vi "New Worker UI.vi"(11 "Starting Name":string) -> (0 "New Project?":bool, 1 "Project":refnum<vi>, 2 "Cancelled?":bool, 3 "New Name":string, 4 "Selected Actions":T1)   [LabVIEW 2022 SP3, in "FlexBlocks Support.lvlib"]
uses:
  FlexBlocks Support.lvlib
  Action Selections.ctl
panel:
  out "Action Diagram":picture
  out "Action Name":string
  out "Info":string
  in  "Actions":T1
  in  "Project Select":string(combo)
  in  "Add To Project":bool
  in  "Cancel":bool
  in  "OK":bool
  # "Enter the name of the new Worker to create:"
  # "Mouseover actions for descriptions."
  # "Unselected actions can later be added to workers by adding the specific case selection back in the Work.vi"
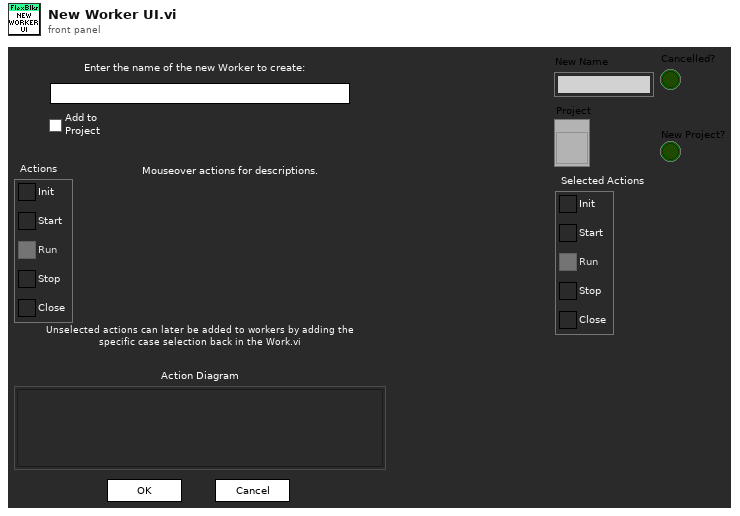
[diagram p1: front panel]
types:
  T1 = typedef "FlexBlocks Support.lvlib/Action Selections.ctl" = cluster{"Init":bool, "Start":bool, "Run":bool, "Stop":bool, "Close":bool}
  T2 = cluster{"Init":bool, "Start":bool, "Run":bool, "Stop":bool, "Close":bool}
  T3 = typedef "FlexBlocks Support.lvlib/Paths.ctl" = cluster{"FlexBlocks":path, "Workers Root":path, "Specialized Editors":path, "Worker Template":path, "SM Template":path, "Read Control Value Vim":path, "Write Indicator Value Vim":path}
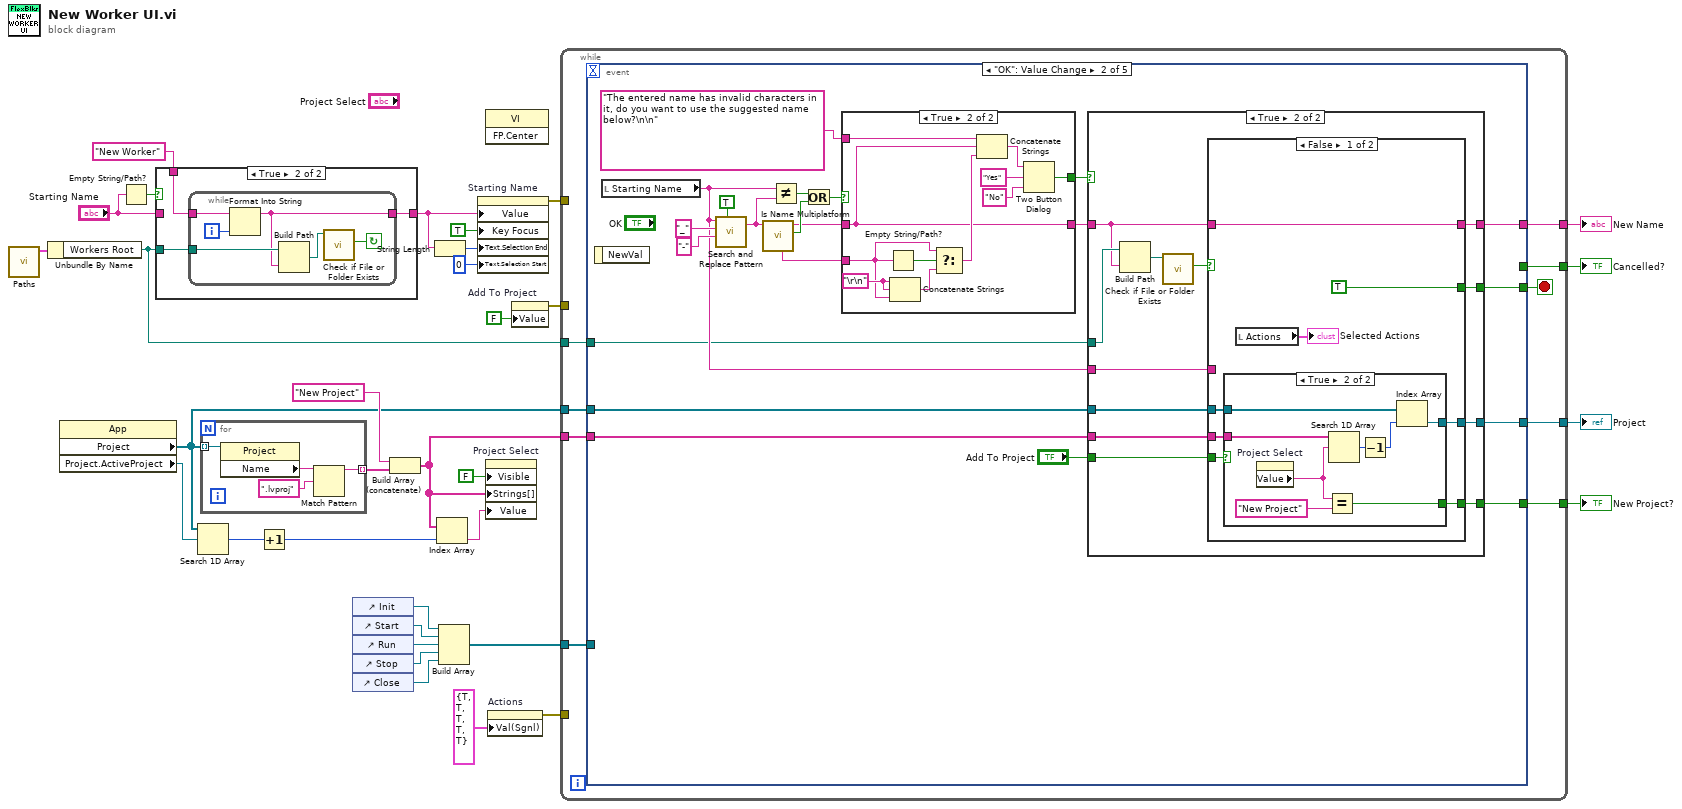
[diagram p0: block diagram]
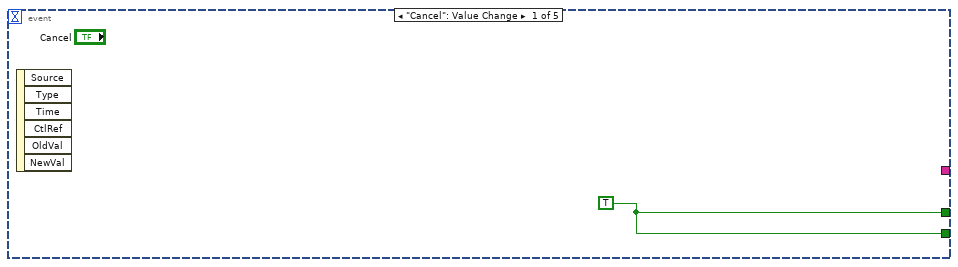
[diagram p2: hidden frame]
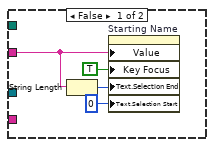
[diagram p3: hidden frame]
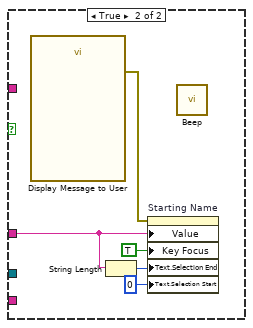
[diagram p5: hidden frame]
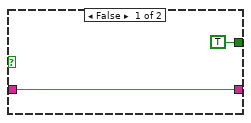
[diagram p6: hidden frame]
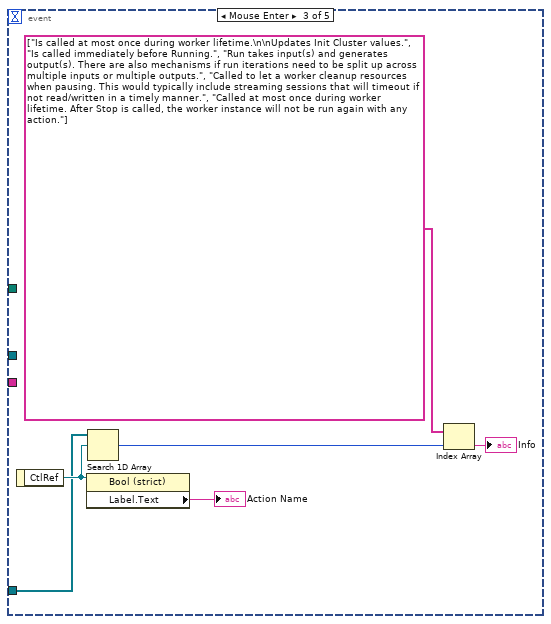
[diagram p7: hidden frame]
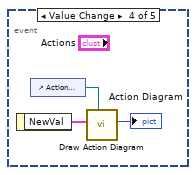
[diagram p8: hidden frame]
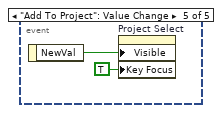
[diagram p9: hidden frame]
diagram:
  n1 = call "Paths.vi"() -> ("Paths"=w18:T3)  [unwired: 11 in]
  n2 = Unbundle By Name(w18) -> ("Workers Root"=w9:path)
  n3 = property class="App"() -> ("Project"=w15:refnum<vi>[], "Project.ActiveProject"=w24:refnum<vi>)  [unwired: 2 in, 2 out]
  n4 = Empty String/Path?(string/path="Starting Name") -> (empty?=w31:bool)
  n5 = case shown="True" w31 {
    tunnel: "Starting Name" -> [w34 _]
    tunnel: w9 -> [_ w37]
    tunnel: [w34 w36] -> w27
    tunnel: "New Worker" -> [_ w35]
    frame False {
    }
    frame True {
      n6 = while {
        tunnel: w37 -> [w42]
        tunnel: [w39] -> w36
        tunnel: w35 -> [w38]
        i -> [w43]
        stop <- w40 continue-if-true
        n7 = Format Into String(initial string=w38, w43) -> (resulting string=w39:string)  [unwired: 2 in, 1 out]
        n8 = Build Path(base path=w42, name or relative path=w39) -> (appended path=w41:path)
        n9 = call <vilib>:"Check if File or Folder Exists.vi"("path"=w41) -> ("file or folder exists?"=w40:bool)  [unwired: 8 in, 2 out]
      }
    }
  }
  n10 = Search 1D Array(1D array=w15, element=w24) -> (index of element=w23:i32)  [unwired: 1 in]
  n11 = for {
    tunnel: w15 -> [w47] mode=indexing
    tunnel: [w44] -> w21 mode=indexing
    n12 = property class="Project"(reference=w47) -> ("Name"=w46:string)  [unwired: 1 in, 2 out]
    n13 = Match Pattern(string=w46, regular expression=".lvproj") -> (before substring=w44:string)  [unwired: 1 in, 3 out]
  }
  n14 = Increment(x=w23) -> (x+1=w19:i32)
  n15 = control-ref of="Init"() -> (w4:refnum<vi>)
  n16 = control-ref of="Start"() -> (w5:refnum<vi>)
  n17 = control-ref of="Run"() -> (w8:refnum<vi>)
  n18 = control-ref of="Stop"() -> (w7:refnum<vi>)
  n19 = control-ref of="Close"() -> (w6:refnum<vi>)
  n20 = Build Array (concatenate)("New Project", w21) -> (w14:string[])
  n21 = String Length(string=w27) -> (length=w29:i32)
  n22 = Index Array(array=w14, index=w19) -> (element=w22:string)
  n23 = Build Array(w4, w5, w8, w7, w6) -> (w3:refnum<vi>[])
  n24 = property on="Starting Name" class="Str"("Value"=w27, "Key Focus"=TRUE, "Text.Selection End"=w29, "Text.Selection Start"=u32 0 ("Text.Selection:Start")) -> (error out=w17:errorcluster)  [unwired: 2 in, 1 out]
  n25 = invoke class="VI" method="FP.Center"() -> ()  [unwired: 3 in, 3 out]
  n26 = property on="Project Select" class="CmbBox"("Visible"=FALSE, "Strings[]"=w14, "Value"=w22) -> ()  [unwired: 2 in, 2 out]
  n27 = property on="Actions" class="Clust (strict)"("Val(Sgnl)"=T2 {"Init"=TRUE, "Start"=TRUE, "Run"=TRUE, "Stop"=TRUE, "Close"=TRUE} ("Value (Signaling)")) -> (error out=w2:errorcluster)  [unwired: 2 in, 1 out]
  n28 = property on="Add To Project" class="Bool (strict)"("Value"=FALSE ("Add To Project")) -> (error out=w16:errorcluster)  [unwired: 2 in, 1 out]
  n29 = while {
    tunnel: w17 -> [_]
    tunnel: w16 -> [_]
    tunnel: w15 -> [w53]
    tunnel: w14 -> [w52]
    tunnel: [w55] -> w13
    tunnel: [w54] -> w12
    tunnel: [w51] -> w11
    tunnel: [w50] -> w10
    tunnel: w9 -> [w49]
    tunnel: w3 -> [w48]
    tunnel: w2 -> [_]
    stop <- w56 stop-if-true
    n30 = event shown="[1] \"OK\": Value Change" {
      selector: _ -> [_ _ _ _ _]
      dyn-events: _ -> [_ _ _ _ _]
      timeout: _ -> [_ _ _ _ _]
      tunnel: [w57 w61 _ _ _] -> w56
      tunnel: [w57 _ _ _ _] -> w55
      tunnel: [_ w65 _ _ _] -> w54
      tunnel: w53 -> [_ w64 _ _ _]
      tunnel: w52 -> [_ w63 _ _ _]
      tunnel: [_ w62 _ _ _] -> w51
      tunnel: [_ w60 _ _ _] -> w50
      tunnel: w49 -> [_ w58 _ _ _]
      tunnel: w48 -> [_ _ w132 _ _]
      event "Cancel": Value Change {
        w57 = TRUE
        n31 = event-data() -> ()  [unwired: 1 in, 6 out]
      }
      event "OK": Value Change {
        n32 = event-data() -> ()  [unwired: 1 in, 1 out]
        n33 = local read "Starting Name"() -> (w59:string)
        n34 = call <vilib>:"Search and Replace Pattern.vi"("string"=w59, "regular expression (\"\")"="_" ("regular expression (\"\")"), "replace string (\"\")"="-" ("replace string (\"\")"), "replace all? (F)"=TRUE) -> ("result string"=w72:string)  [unwired: 1 in, 1 out]
        n35 = call <vilib>:"Is Name Multiplatform.vi"("filename"=w72) -> ("filename had conflict"=w77:bool, "suggested filename"=w76:string, "problem description"=w78:string)  [unwired: 6 in, 2 out]
        n36 = Not Equal?(x=w59, y=w72) -> (x != y?=w70:bool)
        n37 = Or(x=w70, y=w77) -> (x .or. y?=w71:bool)
        n38 = case shown="True" w71 {
          tunnel: w78 -> [_ w122]
          tunnel: w76 -> [w117 w118]
          tunnel: "The entered name has invalid characters in it, do you want to use the suggested name below?\n\n" -> [_ w126]
          tunnel: [TRUE ("T button?") w119] -> w67
          tunnel: [w117 w118] -> w68
          frame False {
          }
          frame True {
            w124 = "\r\n"
            n39 = Empty String/Path?(string/path=w122) -> (empty?=w125:bool)
            n40 = Concatenate Strings(w124, w124, w122) -> (w123:string)
            n41 = Select(t=w122, s=w125, f=w123) -> (s? t:f=w121:string)
            n42 = Concatenate Strings(w126, w118, w121) -> (w120:string)
            n43 = Two Button Dialog(message=w120, 1:"No" ("F button name (\"Cancel\")"), 2:"Yes" ("T button name (\"OK\")")) -> (T button?=w119:bool)
          }
        }
        n44 = case shown="True" w67 {
          tunnel: w68 -> [_ w90]
          tunnel: w58 -> [_ w94]
          tunnel: [_ w91] -> w61
          tunnel: [_ w89] -> w60
          tunnel: w59 -> [w79 w88]
          tunnel: w63 -> [_ w87]
          tunnel: w64 -> [_ w86]
          tunnel: "Add To Project" -> [_ w85]
          tunnel: [_ w84] -> w62
          tunnel: [_ w83] -> w65
          frame False {
            n45 = String Length(string=w79) -> (length=w82:i32)
            n46 = property on="Starting Name" class="Str"("Value"=w79, "Key Focus"=TRUE, "Text.Selection End"=w82, "Text.Selection Start"=u32 0 ("Text.Selection:Start")) -> ()  [unwired: 2 in, 2 out]
          }
          frame True {
            n47 = Build Path(base path=w94, name or relative path=w90) -> (appended path=w93:path)
            n48 = call <vilib>:"Check if File or Folder Exists.vi"("path"=w93) -> ("file or folder exists?"=w92:bool)  [unwired: 8 in, 2 out]
            n49 = case shown="False" w92 {
              tunnel: [TRUE _] -> w91
              tunnel: w90 -> [w101 _]
              tunnel: [w101 _] -> w89
              tunnel: w88 -> [_ w111]
              tunnel: w87 -> [w99 _]
              tunnel: w86 -> [w98 _]
              tunnel: w85 -> [w100 _]
              tunnel: [w97 _] -> w84
              tunnel: [w96 _] -> w83
              frame False {
                n50 = case shown="True" w100 {
                  tunnel: w99 -> [_ w110]
                  tunnel: w98 -> [_ w109]
                  tunnel: [_ w107] -> w97
                  tunnel: [_ w104] -> w96
                  frame False {
                  }
                  frame True {
                    n51 = property on="Project Select" class="CmbBox"() -> ("Value"=w106:string)  [unwired: 2 in, 2 out]
                    n52 = Equal?(x=w106, y="New Project") -> (x = y?=w104:bool)
                    n53 = Search 1D Array(1D array=w110, element=w106) -> (index of element=w108:i32)  [unwired: 1 in]
                    n54 = Decrement(x=w108) -> (x-1=w103:i32)
                    n55 = Index Array(array=w109, index=w103) -> (element=w107:refnum<vi>)
                  }
                }
                n56 = local read "Actions"() -> (→"Selected Actions":T1)
              }
              frame True {
                n57 = call "Display Message to User"() -> ("error out"=w112:errorcluster)  [unwired: 10 in, 1 out]
                n58 = String Length(string=w111) -> (length=w114:i32)
                n59 = property on="Starting Name" class="Str"(error in=w112, "Value"=w111, "Key Focus"=TRUE, "Text.Selection End"=w114, "Text.Selection Start"=u32 0 ("Text.Selection:Start")) -> ()  [unwired: 1 in, 2 out]
                n60 = call <vilib>:"Beep.vi"() -> ()  [unwired: 12 in]
              }
            }
          }
        }
      }
      event Mouse Enter {
        n61 = event-data() -> ("CtlRef"=w133:refnum<vi>)  [unwired: 1 in]
        n62 = property class="Bool (strict)"(reference=w133) -> ("Label.Text"=→"Action Name":string)  [unwired: 1 in, 2 out]
        n63 = Search 1D Array(1D array=w132, element=w133) -> (index of element=w131:i32)  [unwired: 1 in]
        n64 = Index Array(array=string[] ["Is called at most once during worker lifetime.\n\nUpdates Init Cluster values.", "Is called immediately before Running.", "Run takes input(s) and generates output(s). There are also mechanisms if run iterations need to be split up across multiple inputs or multiple outputs.", "Called to let a worker cleanup resources when pausing. This would typically include streaming sessions that will timeout if not read/written in a timely manner.", "Called at most once during worker lifetime. After Stop is called, the worker instance will not be run again with any action."], index=w131) -> (element=→"Info":string)
      }
      event Value Change {
        n65 = event-data() -> ("NewVal"=w137:T1)  [unwired: 1 in]
        n66 = control-ref of="Action Diagram"() -> (w135:refnum<vi>)
        n67 = call "Draw Action Diagram.vi"("Diagram Ref"=w135, "Actions"=w137) -> ("Action Diagram"=→"Action Diagram":picture)  [unwired: 9 in]
      }
      event "Add To Project": Value Change {
        n68 = event-data() -> ("NewVal"=w138:bool)  [unwired: 1 in]
        n69 = property on="Project Select" class="CmbBox"("Visible"=w138, "Key Focus"=TRUE) -> ()  [unwired: 2 in, 2 out]
      }
    }
  }
  "Cancelled?" <- w13
  "New Name" <- w10
  "Project" <- w11
  "New Project?" <- w12
